vi "Get Path To Private Data Control And Parent Class.vi"(8 "error in (no error)":errorcluster, 11 "Class":path) -> (0 "error out":errorcluster, 1 "Private Data Control":path, 2 "Parent":path)   [LabVIEW 2017, in "Composition.lvlib"]
doc: "Reads the path to the private data control and the parent class of the specified class."
uses:
  Composition.lvlib
  <vilib>/Utility/lvfile.llb/LVFileType.ctl
  <vilib>/Utility/lvfile.llb/NI_FileType.lvlib
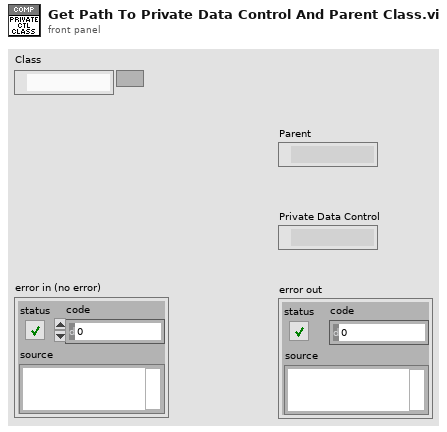
[diagram p1: front panel]
types:
  T1 = typedef "NI_FileType.lvlib/LVFileType.ctl" = enum32{"Invalid file", "Unknown type", "Instrument", "Control", "Polymorphic VI", "Project", "Library", "LVClass", "XControl", "XNode", "Shared library", ".NET assembly", "ActiveX interface", "CIN", "Run-time menu", "Palette menu", "Help file", "LLB", "XNode Edit Dependency", "Class Private Data Control", "Statechart", "MathScript .m file", "Ladder Diagram", "LVLibp", "XNode Build Dependency"}
  T2 = cluster{"path":path, "delimited name":string, "type":T1, "iState":u32, "iStyle":u16, "wStyle":u16, "buttons":u16, "viflags":u32, "viflags2":u32, "links":u32[]}[]
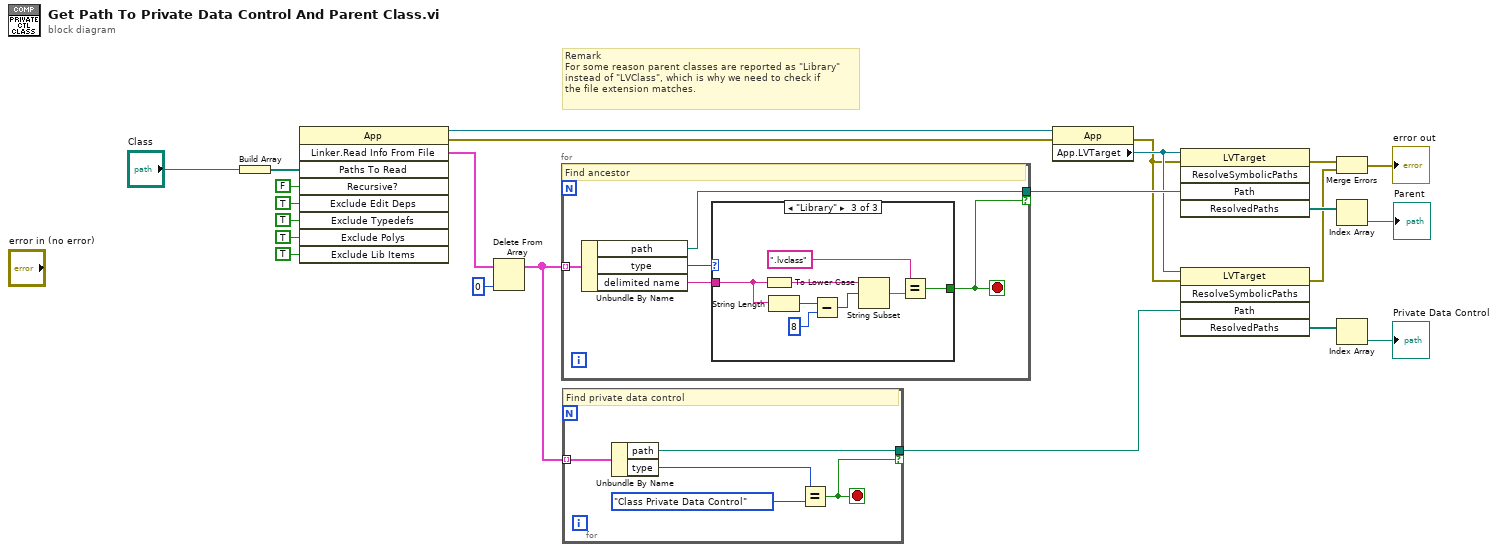
[diagram p0: block diagram]
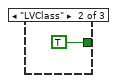
[diagram p3: hidden frame]
diagram:
  # "Remark\nFor some reason parent classes are reported as \"Library\"\ninstead of \"LVClass\", which is why we need to check if\nthe file extension matches."
  n1 = Build Array("Class") -> (w23:path[])
  n2 = invoke class="App" method="Linker.Read Info From File"("Paths To Read"=w23, "Recursive?"=FALSE, "Exclude Edit Deps"=TRUE ("Exclude Edit Time Dependencies"), "Exclude Typedefs"=TRUE, "Exclude Polys"=TRUE ("Exclude Poly VIs"), "Exclude Lib Items"=TRUE ("Exclude Unused Library Items")) -> (reference out=w16:refnum<vi>, error out=w15:errorcluster, "Linker.Read Info From File"=w13:T2)  [unwired: 3 in, 6 out]
  n3 = Delete From Array(array=w13, index=0) -> (array with subset deleted=w12:T2)  [unwired: 1 in, 1 out]
  n4 = for {
    tunnel: w12 -> [w28] mode=indexing
    tunnel: [w26] -> w14 if=w24
    stop <- w24 stop-if-true
    # "Find ancestor"
    n5 = Unbundle By Name(w28) -> ("path"=w26:path, "type"=w27:T1, "delimited name"=w25:string)
    n6 = case shown="\"Library\"" w27 {
      tunnel: [_ TRUE w30] -> w24
      tunnel: w25 -> [_ _ w35]
      frame Default {
      }
      frame "LVClass" {
      }
      frame "Library" {
        n7 = To Lower Case(string=w35) -> (all lower case string=w37:string)
        n8 = String Length(string=w35) -> (length=w36:i32)
        n9 = Subtract(x=w36, y=8) -> (x-y=w34:i32)
        n10 = String Subset(string=w37, offset (0)=w34) -> (substring=w32:string)  [unwired: 1 in]
        n11 = Equal?(x=".lvclass", y=w32) -> (x = y?=w30:bool)
      }
    }
  }
  n12 = for {
    tunnel: w12 -> [w42] mode=indexing
    tunnel: [w41] -> w11 if=w38
    stop <- w38 stop-if-true
    # "Find private data control"
    n13 = Unbundle By Name(w42) -> ("path"=w41:path, "type"=w40:T1)
    n14 = Equal?(x=w40, y=LVFileType."Class Private Data Control") -> (x = y?=w38:bool)
  }
  n15 = property class="App"(reference=w16, error in=w15) -> (error out=w7:errorcluster, "App.LVTarget"=w8:refnum<vi>)  [unwired: 1 out]
  n16 = invoke class="LVTarget" method="ResolveSymbolicPaths"(reference=w8, error in=w7, "Path"=w14) -> (error out=w4:errorcluster, "ResolvedPaths"=w10:path[])  [unwired: 2 in, 3 out]
  n17 = invoke class="LVTarget" method="ResolveSymbolicPaths"(reference=w8, error in=w7, "Path"=w11) -> (error out=w3:errorcluster, "ResolvedPaths"=w5:path[])  [unwired: 2 in, 3 out]
  n18 = Merge Errors(w4, w3) -> (→"error out":errorcluster)
  n19 = Index Array(array=w10) -> (element=→"Parent":path)  [unwired: 1 in]
  n20 = Index Array(array=w5) -> (element=→"Private Data Control":path)  [unwired: 1 in]
